vi "Create All Message Queues.vi"(8 "error in (no error)":errorcluster) -> (0 "error out":errorcluster, 3 "Message queues out":T1)   [LabVIEW 2021, in "dcvmMessageQueue.lvlib"]
doc: "This VI creates and initializes all the message queues for your application. If your application requires more than one message queue, right-click the \"Message Queues\" constant above and select Open Type Def. Add the new Message Queue(s) to the type definition, then initialize them in this VI."
uses:
  dcvmMessageQueue.lvlib
  controls/Message Queues.ctl
  controls/Message Data.ctl
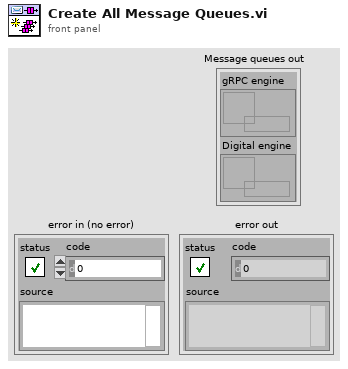
[diagram p1: front panel]
types:
  T1 = typedef "dcvmMessageQueue.lvlib/Message Queues.ctl" = cluster{"gRPC engine":refnum<queue>, "Digital engine":refnum<queue>}
  T2 = typedef "dcvmMessageQueue.lvlib/Message Data.ctl" = cluster{"Action":string, "Value":variant}
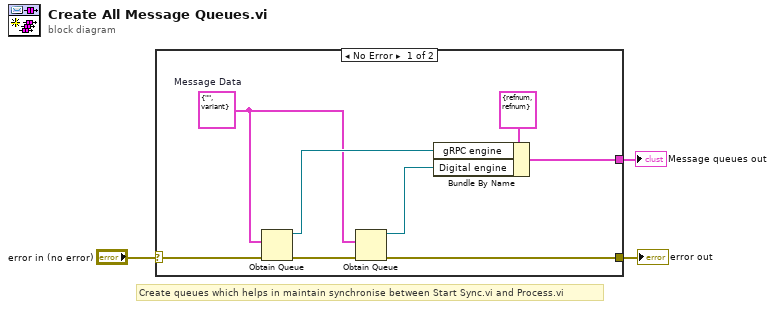
[diagram p0: block diagram]
diagram:
  # "Create queues which helps in maintain synchronise between Start Sync.vi and Process.vi"
  n1 = case shown="No Error" "error in (no error)" {
    selector: "error in (no error)" -> [w6 w12]
    tunnel: [w4 w12] -> w3
    tunnel: [w10 _] -> w2
    frame No Error {
      w7 = T2 {"Action"="", "Value"=variant}  # Message Data
      n2 = Obtain Queue(element data type=w7, error in (no error)=w6) -> (queue out=w9:refnum<queue>, error out=w5:errorcluster)  [unwired: 3 in, 1 out]
      n3 = Obtain Queue(element data type=w7, error in (no error)=w5) -> (queue out=w8:refnum<queue>, error out=w4:errorcluster)  [unwired: 3 in, 1 out]
      n4 = Bundle By Name(cluster=T1 {"gRPC engine"=refnum, "Digital engine"=refnum} ("Message Queues"), "gRPC engine"=w9, "Digital engine"=w8) -> (w10:T1)
    }
    frame Error {
    }
  }
  "Message queues out" <- w2
  "error out" <- w3
